vi "Revision Query.vi"(8 "error in (no error)":errorcluster, 11 "CS++DMM in":refnum<class "CS++DMM.lvclass">) -> (0 "error out":errorcluster, 1 "Firmware Revision":string, 2 "Driver Revision":string, 3 "CS++DMM out":refnum<class "CS++DMM.lvclass">)   [LabVIEW 2013, in "CS++DMM.lvlib" / "CS++DMM.lvclass"]
uses:
  CS++DMM.lvclass
  Core/Actors/CS++DeviceActor/CS++DeviceActor.lvclass
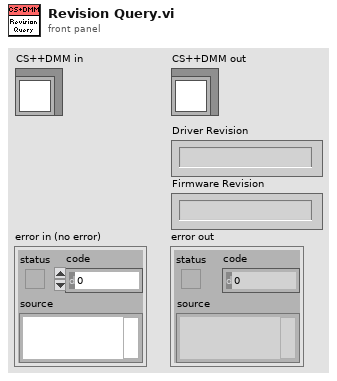
[diagram p1: front panel]
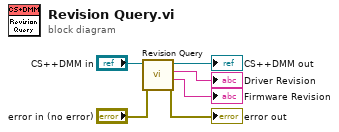
[diagram p0: block diagram]
diagram:
  n1 = call-parent "Revision Query.vi"("error in (no error)"="error in (no error)", "CS++DeviceActor in"="CS++DMM in") -> ("error out"=→"error out":errorcluster, "Firmware Revision"=→"Firmware Revision":string, "Driver Revision"=→"Driver Revision":string, "CS++DeviceActor out"=→"CS++DMM out":refnum<class "CS++DMM.lvclass">)  [unwired: 6 in]
